vi "variant data type.vi"(9 "data":variant, 10 "data_unit":T1=enum."string") -> (0 "Date/Time":string, 1 "Numeric (DBL)":dbl format="%#_6f", 2 "Numeric (SGL)":sgl format="%#_6f", 3 "Numeric (I32)":i32, 4 "bool":bool, 5 "String":string)   [LabVIEW 2020]
uses:
  controls/data type.ctl
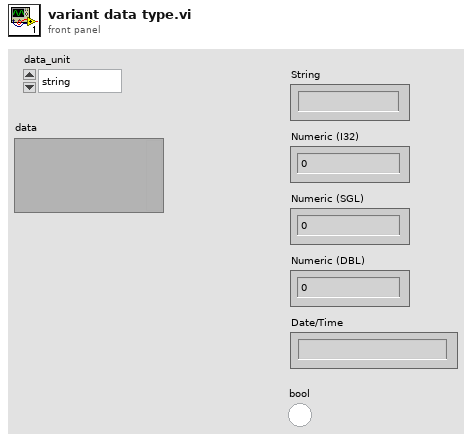
[diagram p1: front panel]
types:
  T1 = typedef "data type.ctl" = enum16{"bool", "string", "I32", "SGL", "DBL", "Date/Time"}
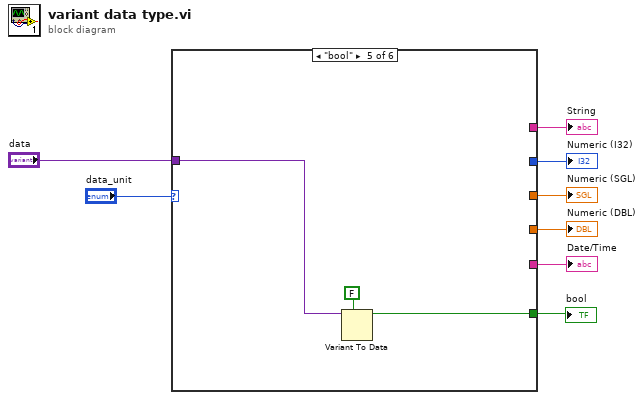
[diagram p0: block diagram]
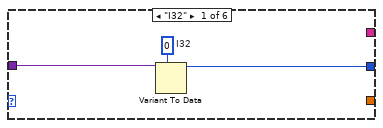
[diagram p2: hidden frame]
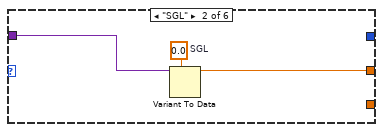
[diagram p3: hidden frame]
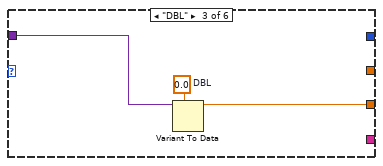
[diagram p4: hidden frame]
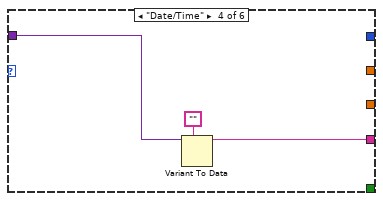
[diagram p5: hidden frame]
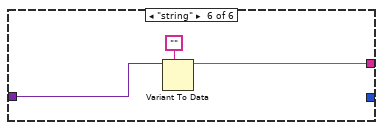
[diagram p6: hidden frame]
diagram:
  n1 = case shown="\"bool\"" "data_unit" {
    tunnel: [_ _ _ _ _ w25] -> w8
    tunnel: [w11 _ _ _ _ _] -> w7
    tunnel: [_ w14 _ _ _ _] -> w6
    tunnel: [_ _ w17 _ _ _] -> w5
    tunnel: [_ _ _ w20 _ _] -> w4
    tunnel: "data" -> [w9 w12 w15 w18 w23 w24]
    tunnel: [_ _ _ _ w21 _] -> w2
    frame "I32" {
      w10 = 0  # I32
      n2 = Variant To Data(type=w10, Variant=w9) -> (data=w11:i32)  [unwired: 1 in, 1 out]
    }
    frame "SGL" {
      w13 = sgl 0.0  # SGL
      n3 = Variant To Data(type=w13, Variant=w12) -> (data=w14:sgl)  [unwired: 1 in, 1 out]
    }
    frame "DBL" {
      w16 = 0.0  # DBL
      n4 = Variant To Data(type=w16, Variant=w15) -> (data=w17:dbl)  [unwired: 1 in, 1 out]
    }
    frame "Date/Time" {
      n5 = Variant To Data(type="", Variant=w18) -> (data=w20:string)  [unwired: 1 in, 1 out]
    }
    frame "bool" {
      n6 = Variant To Data(type=FALSE, Variant=w23) -> (data=w21:bool)  [unwired: 1 in, 1 out]
    }
    frame "string" {
      n7 = Variant To Data(type="" ("String"), Variant=w24) -> (data=w25:string)  [unwired: 1 in, 1 out]
    }
  }
  "String" <- w8
  "Numeric (I32)" <- w7
  "Numeric (SGL)" <- w6
  "Numeric (DBL)" <- w5
  "Date/Time" <- w4
  "bool" <- w2
